vi "TCP-read.vi"(3 "timeout (5000)":i32=3000, 4 "error in (no error)":errorcluster, 5 "connection ID":refnum<k5>) -> (0 "error out":errorcluster, 1 "data out":string, 2 "keyword":string)   [LabVIEW 2019]
panel:
  out "basic_answer":string
  out "number":string
  out "nBytes":i32
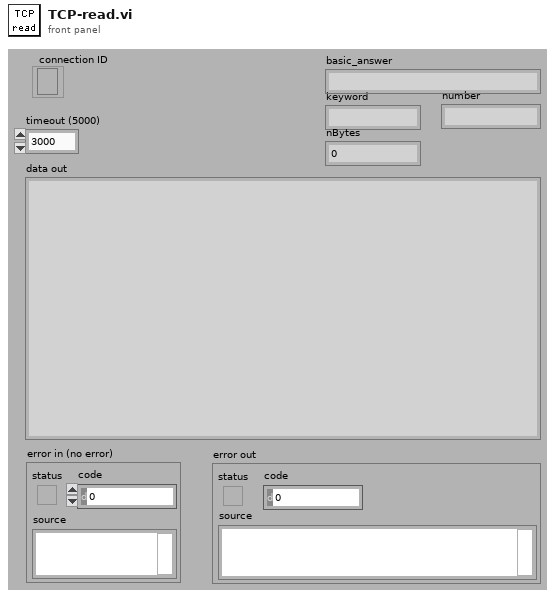
[diagram p1: front panel]
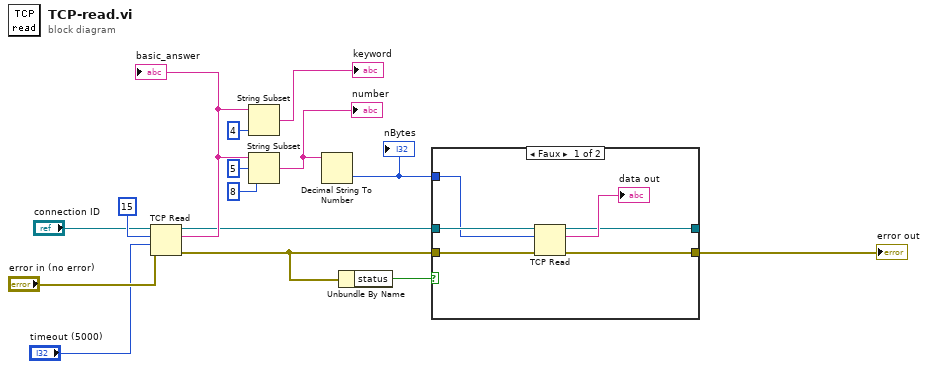
[diagram p0: block diagram]
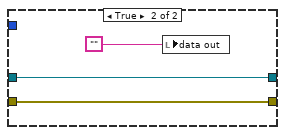
[diagram p2: hidden frame]
diagram:
  n1 = TCP Read(connection ID="connection ID", bytes to read=15, error in (no error)="error in (no error)", 9:"timeout (5000)") -> (connection ID out=w8:refnum<k5>, data out=w12:string, error out=w6:errorcluster)  [unwired: 1 in]
  "basic_answer" <- w12
  n2 = String Subset(string=w12, length (rest)=4 ("length (rest)")) -> (substring=→"keyword":string)  [unwired: 1 in]
  n3 = String Subset(string=w12, offset (0)=5, length (rest)=8 ("length (rest)")) -> (substring=w9:string)
  "number" <- w9
  n4 = Decimal String To Number(string=w9) -> (number=w5:i32)  [unwired: 2 in, 1 out]
  "nBytes" <- w5
  n5 = Unbundle By Name(w6) -> ("status"=w7:bool)
  n6 = case shown="Faux" w7 {
    tunnel: w8 -> [w21 w23]
    tunnel: w6 -> [w20 w24]
    tunnel: w5 -> [w18 _]
    tunnel: [w17 w24] -> w4
    tunnel: [w16 w23] -> _
    frame False {
      n7 = TCP Read(connection ID=w21, bytes to read=w18, error in (no error)=w20) -> (connection ID out=w16:refnum<k5>, data out=→"data out":string, error out=w17:errorcluster)  [unwired: 2 in]
    }
    frame True {
      n8 = local write "data out"("") -> ()
    }
  }
  "error out" <- w4
